vi "Global_CMD.vi"() -> ()   [LabVIEW 2017, in "Claw.lvlib"]
uses:
  startup.rtexe/Claw.lvlib
  startup.rtexe/CLUSTER_Two Motor Input.ctl
panel:
  in  "CMD_Disable_Claw":bool
  in  "CMD_Claw_Speeds":T1
  in  "CMD_Claw_Piston":bool
  # "The Names of the Data items in the Global Variable MUST describe who the Single Writer is\nNaming Convention for Command Globals is:   \n\nCMD_SubSystem_Data Name\nExample:\nCMD_Drive_Mode\nCMD_Hopper_Fire Ball"
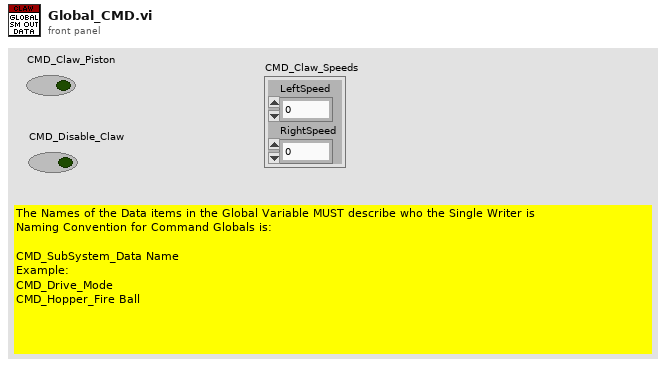
[diagram p1: front panel]
types:
  T1 = typedef "CLUSTER_Two Motor Input.ctl" = cluster{"LeftSpeed":dbl, "RightSpeed":dbl}
diagram:
